vi "MT ASK Transmitter.vi"() -> ()   [LabVIEW 2015]
uses:
  <vilib>/addons/Modulation/Digital/Support/Common/Validators/mod_Generate Bits Validate.vi
  <vilib>/addons/Modulation/Analog/support/mod_Set Error Source.vi
  <vilib>/addons/Modulation/Digital/General/subVIs/mod_Generate Bits PN Sequence.vi
  <vilib>/addons/Modulation/Digital/Support/Common/Validators/mod_Generate Filter Coefficients Validate.vi
  <vilib>/addons/Modulation/Digital/General/subVIs/mod_Generate Filter Coefficients.vi
  <vilib>/addons/Modulation/Analog/MT Upconvert Baseband (Real).vi
  <vilib>/addons/Modulation/Digital/General/MT Generate Bits (Galois, PN Order).vi
  <vilib>/addons/Modulation/Digital/General/MT Generate ASK system parameters (M).vi
  <instrlib>/niUSRP/niUSRP Write Tx Data (CDB WDT).vi
  <vilib>/addons/Modulation/niDMT.lvlib
  <vilib>/addons/Modulation/niAMT.lvlib
panel:
  in  "Tab Control 3":enum32{"Page 1", "Page 2"}(tab)
  out "error out":errorcluster
  out "coerced IQ rate":dbl=100000.0 format="%#_6p"
  out "coerced gain":dbl format="%#_6f"
  out "coerced carrier frequency":dbl=100000.0 format="%#_6p"
  in  "Tab Control 2":enum32{"Page 1", "Page 2"}(tab)
  in  "device names":refnum<k15>
  in  "IQ rate":dbl=100000.0 format="%#_6p"
  in  "gain":dbl format="%#_6f"
  in  "Carrier Frequency":dbl=100000.0 format="%#_6p"
  in  "Active Antenna":string
  in  "M-ASK":i32=2
  in  "pulse shaping filter (none)":T1(ring) caption="Pulse Shaping Filter"
  in  "symbol rate (Hz)":dbl=1.0 caption="Symbol Rate" format="%.2f"
  in  "Stop":bool
  in  "Tab Control":enum32{"Graphs", "Constellation"}(tab)
  out "Modulating":dbl[](graph)
  out "Modulated":waveform(dbl)(graph)
  out "XY Graph":T2(graph)
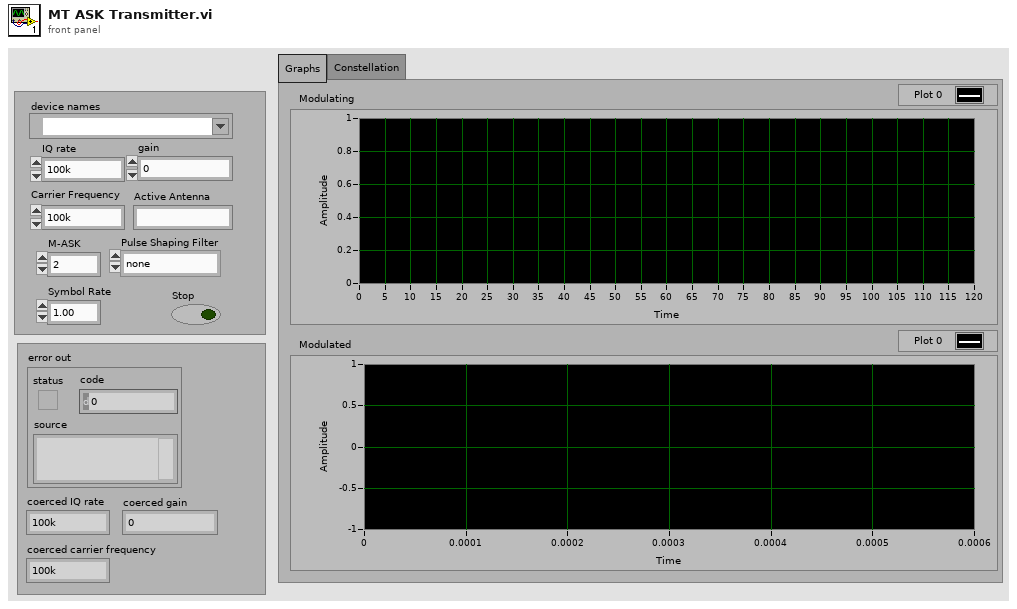
[diagram p1: front panel]
types:
  T1 = enum16{"none", "Raised Cosine", "Root Raised Cos", "Gaussian"}
  T2 = cluster{"constellation":dbl[], "oversampled data":dbl[]}[]
  T3 = enum16{"FSK", "PSK", "QAM", "MSK", "PAM", "ASK", "CPM"}
  T4 = cluster{"samples per symbol (16)":i32, "symbol map":cdb[]}
  T5 = typedef "niAMT.lvlib/Complex Data Waveform.ctl" = cluster{"t0":dbl, "dt":dbl, "Y":cdb[]}
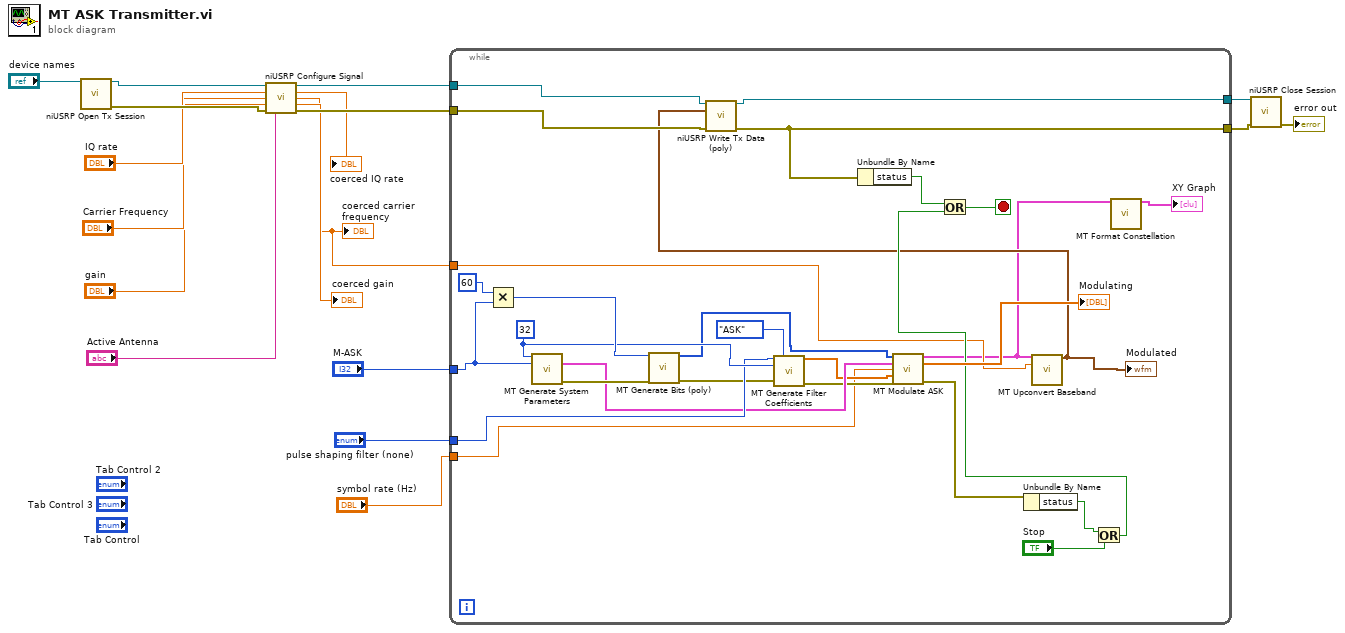
[diagram p0: block diagram]
diagram:
  n1 = call <instrlib>:"niUSRP Open Tx Session.vi"("device names"="device names") -> ("session handle out"=w14:refnum<k15>, "error out"=w18:errorcluster)  [unwired: 13 in]
  n2 = call <instrlib>:"niUSRP Configure Signal.vi"("session handle"=w14, "IQ rate"="IQ rate", "carrier frequency"="Carrier Frequency", "gain"="gain", "error in (no error)"=w18, "active antenna"="Active Antenna") -> ("session handle out"=w13:refnum<k15>, "coerced IQ rate"=→"coerced IQ rate":dbl, "coerced carrier frequency"=w2:dbl, "coerced gain"=→"coerced gain":dbl, "error out"=w17:errorcluster)  [unwired: 5 in]
  "coerced carrier frequency" <- w2
  n3 = while {
    tunnel: w17 -> [w46]
    tunnel: [w26] -> w16
    tunnel: w13 -> [w45]
    tunnel: [w44] -> w12
    tunnel: "M-ASK" -> [w42]
    tunnel: "pulse shaping filter (none)" -> [w38]
    tunnel: "symbol rate (Hz)" -> [w32]
    tunnel: w2 -> [w22]
    stop <- w23 stop-if-true
    w39 = 32 ("samples per symbol (16)")
    n4 = Multiply(x=60, y=w42) -> (x*y=w40:i32)
    n5 = call-poly <vilib>:"MT Generate System Parameters.vi"("samples per symbol (16)"=w39, "M-ASK (2)"=w42) -> ("ASK system parameters"=w35:T4, "error out"=w43:errorcluster)  [unwired: 11 in, 1 out]
    n6 = call-poly <vilib>:"MT Generate Bits (poly).vi"("total bits (128)"=w40, "error in (no error)"=w43) -> ("output bit stream"=w31:i8[], "error out"=w37:errorcluster)  [unwired: 11 in, 1 out]
    n7 = call <vilib>:"MT Generate Filter Coefficients.vi"("pulse shaping filter (none)"=w38, "modulation type"=T3."ASK", "pulse shaping samples per symbol (16)"=w39, "error in (no error)"=w37) -> ("pulse shaping filter coefficients"=w33:dbl[], "error out"=w34:errorcluster)  [unwired: 9 in, 1 out]
    n8 = call <vilib>:"MT Modulate ASK.vi"("input bit stream"=w31, "ASK system parameters"=w35, "symbol rate (Hz)"=w32, "pulse shaping filter coefficients"=w33, "error in (no error)"=w34) -> ("output complex waveform"=w20:T5, "symbols out"=→"Modulating":cdb[], "error out"=w28:errorcluster)  [unwired: 8 in]
    n9 = Unbundle By Name(w28) -> ("status"=w30:bool)
    n10 = call-poly <vilib>:"MT Upconvert Baseband.vi"("baseband waveform (complex)"=w20, "carrier frequency (Hz)"=w22) -> ("passband waveform"=w21:waveform(dbl))  [unwired: 12 in, 1 out]
    "Modulated" <- w21
    n11 = call-poly <instrlib>:"niUSRP Write Tx Data (poly).vi"("session handle"=w45, "data"=w21, "error in (no error)"=w46) -> ("session handle out"=w44:refnum<k15>, "error out"=w26:errorcluster)  [unwired: 11 in]
    n12 = Unbundle By Name(w26) -> ("status"=w25:bool)
    n13 = Or(x=w30, y="Stop") -> (x .or. y?=w24:bool)
    n14 = Or(x=w25, y=w24) -> (x .or. y?=w23:bool)
    n15 = call <vilib>:"MT Format Constellation.vi"("waveform"=w20) -> ("constellation graph"=→"XY Graph":T2)  [unwired: 13 in, 1 out]
  }
  n16 = call <instrlib>:"niUSRP Close Session.vi"("session handle"=w12, "error in (no error)"=w16) -> ("error out"=→"error out":errorcluster)  [unwired: 13 in]
